vi "Convert Filter INI String to Cluster.vi"(11 "INI String":string) -> (3 "Filter Info":T1={"Filter Column"=enum."Description", "Filter Type"=enum."Contains", "Filter Value"="", "New Data?"=FALSE, "Enabled?"=FALSE})   [LabVIEW 2023, in "VI Properties Editor.lvlib"]
doc: "Converts a filter as <B>INI String</B> to a cluster."
uses:
  VI Properties Editor.lvlib
  CTLs/Filter Info.ctl
  CTLs/Column Name.ctl
  CTLs/Filter Type.ctl
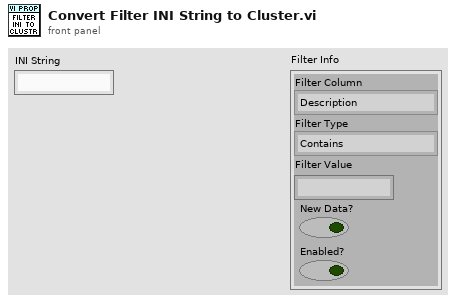
[diagram p1: front panel]
types:
  T1 = typedef "VI Properties Editor.lvlib/Filter Info.ctl" = cluster{"Filter Column":T2, "Filter Type":T3, "Filter Value":string, "New Data?":bool, "Enabled?":bool}
  T2 = typedef "VI Properties Editor.lvlib/Column Name.ctl" = enum16{"Name", "Path", "Type", "Window Title", "Description", "Help Path", "Help Tag", "Custom Title?", "Reentrant?", "Inlined?"}
  T3 = typedef "VI Properties Editor.lvlib/Filter Type.ctl" = enum16{"Contains", "Equals", "Starts with", "Ends with", "Does not contain", "Does not equal", "Is empty", "Is not empty"}
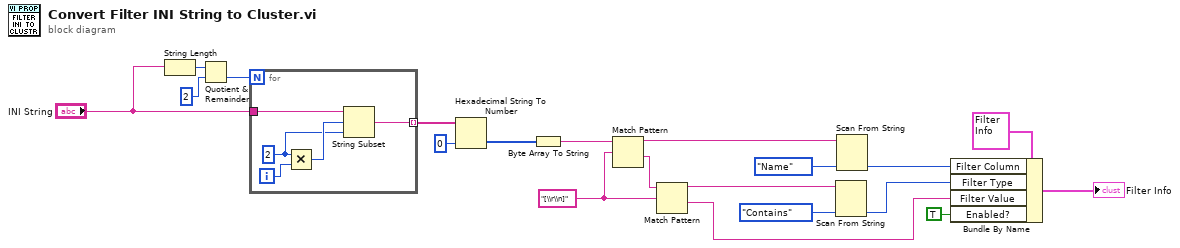
[diagram p0: block diagram]
diagram:
  w12 = "[\\r\\n]" ("regular expression")
  n1 = String Length(string="INI String") -> (length=w19:i32)
  n2 = Quotient & Remainder(x=w19, y=2) -> (floor(x/y)=w17:i32)  [unwired: 1 out]
  n3 = for {
    N: w17 -> [_]
    tunnel: "INI String" -> [w25]
    tunnel: [w21] -> w16 mode=indexing
    i -> [w24]
    w22 = 2 ("x")
    n4 = Multiply(x=w22, y=w24) -> (x*y=w23:i32)
    n5 = String Subset(string=w25, offset (0)=w23, length (rest)=w22) -> (substring=w21:string)
  }
  n6 = Hexadecimal String To Number(string=w16, default (0uL)=u8 0 ("default (0 U32)")) -> (number=w15:u8[])  [unwired: 1 in, 1 out]
  n7 = Byte Array To String(unsigned byte array=w15) -> (string=w14:string)
  n8 = Match Pattern(string=w14, regular expression=w12) -> (before substring=w9:string, after substring=w13:string)  [unwired: 1 in, 2 out]
  n9 = Match Pattern(string=w13, regular expression=w12) -> (before substring=w8:string, after substring=w3:string)  [unwired: 1 in, 2 out]
  n10 = Scan From String(input string=w8, default 1=Filter_Type."Contains" ("Filter Type")) -> (output 1=w4:T3)  [unwired: 3 in, 3 out]
  n11 = Scan From String(input string=w9, default 1=Column_Name."Name" ("Filter Column")) -> (output 1=w6:T2)  [unwired: 3 in, 3 out]
  n12 = Bundle By Name(cluster=T1 {"Filter Column"=enum."Description", "Filter Type"=enum."Contains", "Filter Value"="", "New Data?"=FALSE, "Enabled?"=FALSE} ("Filter Info"), "Filter Column"=w6, "Filter Type"=w4, "Filter Value"=w3, "Enabled?"=TRUE) -> (→"Filter Info":T1)
